vi "readStdErr.vi"(8 "error in (no error)":errorcluster, 9 "Bytes to read":u32=10 min=1, 10 "Pipe buffer size":u32=30 min=4, 11 "STD IN/OUT":u32(ring)=4294967284 items=["STD_OUTPUT_HANDLE"=4294967285, "STD_ERROR_HANDLE"=4294967284]) -> (2 "Numeric":i32, 3 "Out":string)   [LabVIEW 2013]
uses:
  kernel32.dll
panel:
  out "error out":errorcluster
  in  "stop":bool
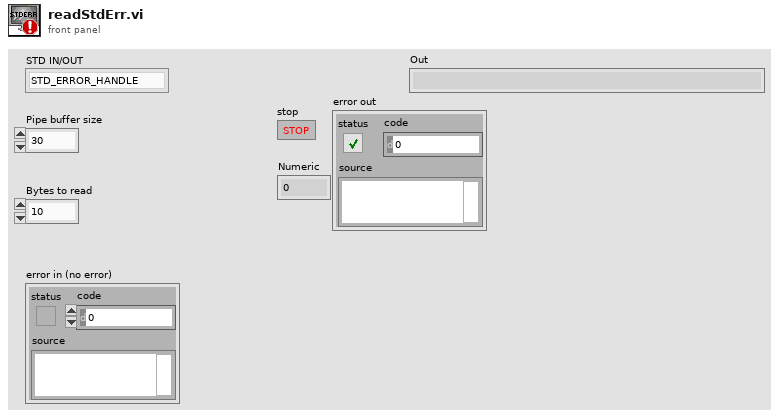
[diagram p1: front panel]
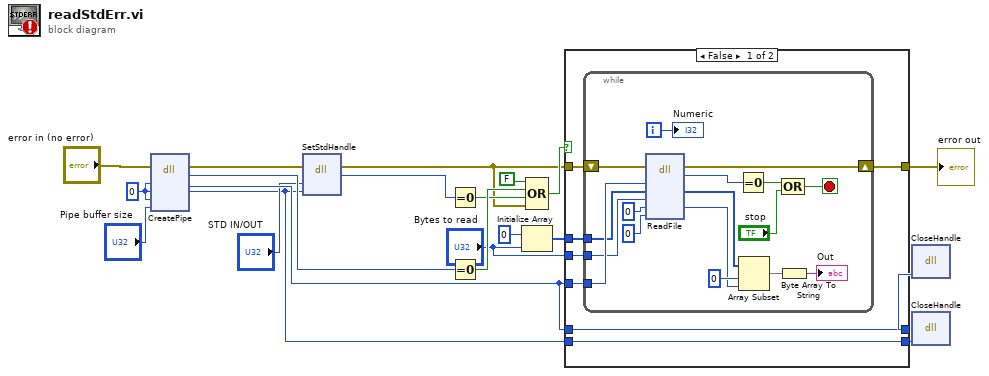
[diagram p0: block diagram]
diagram:
  w20 = u64 0 ("hReadPipe")
  n1 = dll-call lib="kernel32.dll" fn="CreatePipe"(error in="error in (no error)", "hReadPipe"=w20, "hWritePipe"=w20, "lpPipeAttributes"=w20, "nSize"="Pipe buffer size") -> (error out=w5:errorcluster, "BOOL"=w19:i32, "hReadPipe"=w12:u64, "hWritePipe"=w2:u64)  [unwired: 4 in, 1 out]
  n2 = dll-call lib="kernel32.dll" fn="SetStdHandle"(error in=w5, "nStdHandle"="STD IN/OUT", "hHandle"=w2) -> (error out=w3:errorcluster, "BOOL"=w17:i32)  [unwired: 4 in, 1 out]
  n3 = Equal To 0?(x=w17) -> (x = 0?=w16:bool)
  n4 = Equal To 0?(x=w19) -> (x = 0?=w18:bool)
  n5 = Initialize Array(u8 0 ("element"), "Bytes to read") -> (w9:u8[])
  n6 = Compound Arithmetic op=OR(FALSE ("value"), w18, w16, w3) -> (w4:bool)
  n7 = case shown="False" w4 {
    tunnel: w3 -> [w25 w45]
    tunnel: [w27 w47] -> w14
    tunnel: w12 -> [w27 w47]
    tunnel: [w26 w46] -> w13
    tunnel: w2 -> [w26 w46]
    tunnel: w12 -> [w24 _]
    tunnel: w9 -> [w23 _]
    tunnel: "Bytes to read" -> [w22 _]
    tunnel: [w21 w45] -> w1
    frame False {
      n8 = while {
        shift-right: [w41] -> w21
        shift-left: w25 -> [w42]
        tunnel: w24 -> [w40]
        tunnel: w23 -> [w39]
        tunnel: w22 -> [w38]
        i -> [w28]
        stop <- w43 stop-if-true
        n9 = dll-call lib="kernel32.dll" fn="ReadFile"(error in=w42, "hFile"=w40, "lpBuffer"=w39, "nNumberOfBytesToRead"=w38, "lpNumberOfBytesRead"=u32 0, "lpOverlapped"=u64 0) -> (error out=w41:errorcluster, "BOOL"=w30:i32, "lpBuffer"=w35:u8[], "lpNumberOfBytesRead"=w33:u32)  [unwired: 5 in, 1 out]
        n10 = Equal To 0?(x=w30) -> (x = 0?=w29:bool)
        n11 = Array Subset(array=w35, index=0, length=w33) -> (w32:u8[])
        n12 = Byte Array To String(unsigned byte array=w32) -> (string=→"Out":string)
        n13 = Compound Arithmetic op=OR(w29, "stop") -> (w43:bool)
        "Numeric" <- w28
      }
    }
    frame True {
    }
  }
  "error out" <- w1
  n14 = dll-call lib="kernel32.dll" fn="CloseHandle"("hObject"=w14) -> ()  [unwired: 5 in, 2 out]
  n15 = dll-call lib="kernel32.dll" fn="CloseHandle"("hObject"=w13) -> ()  [unwired: 5 in, 2 out]
